vi "asap_rt_loop.vi"(4 "ASAP config":T1={"Calibration data"={"T1"=[], "K1"=[], "T2"=[], "K2"=[]}, "Block size"=0, "Tasks"={"Analog Input"="", "Counters"=[], "Digital out"=""}, "Light enables"=[], "Demodulator table"=[[[0.7378876894649258, 0.0906125472597644, -0.6039607285908369, -0.9832772754191942, -0.8493406206796001, -0.27206330946071283, 0.4472261971995385, 0.9330716049510009, 0.9318702757288254, 0.44424928196195224, -0.27526191405131173, -0.8510913000722428, -0.9826662061933111, -0.6013068779842613, 0.09392391656034481, 0.7401281017410278, 0.999998617584093], [0.9593453970107514, 0.1749709233028358, -0.8033628936873337, -0.8911502339509838, 0.008923213624955564, 0.8991050710898453, 0.7926080184909147, -0.19251348121496464, -0.9642293036540662, -0.6670744875896746, 0.36954793309667006, 0.9965178637479297, 0.5188245350812338, -0.5339978733406581, -0.9948712031832995, -0.3529066352920418, 0.6802631564678894]], [[0.6950304448649641, 0.029259796336992095, -0.6517839440467688, -0.9926080898406189, -0.8153085153483962, -0.21243243641618328, 0.5013295857114554, 0.9534065050307919, 0.907822232196422, 0.3883709446578477, -0.3338030496133024, -0.8817378051772073, -0.969421151739755, -0.5510839461787943, 0.15490925101319897, 0.7800425818962478, 0.9980075966531081], [0.9381204165433596, 0.10815294018097958, -0.8417045890860233, -0.8585129793585211, 0.07636026142185437, 0.9265863741042095, 0.749669912334455, -0.25827310590600655, -0.979914371470141, -0.615297735575794, 0.43139076953297817, 0.9998725601934042, 0.45997233240039587, -0.5898179378997009, -0.9857812880942376, -0.2889831231211053, 0.728159563799897]], [[-0.6523106754624476, 0.028565353817145308, 0.6945307778513148, 0.9979635224154992, 0.7804771064006715, 0.15559556021784737, -0.5505040934388046, -0.969250428253351, -0.8820653255595329, -0.33445785406592654, 0.38773065238112236, 0.9075306732447919, 0.953615867977217, 0.5019305868317728, -0.2117535089882616, -0.814906049621952, -0.9926921657471056], [-0.8972537749411549, -0.004712231334943897, 0.8930529304466017, 0.800848121012319, -0.17911548107307929, -0.9605254010675951, -0.6771705448338604, 0.3568436305984995, 0.9952883311784719, 0.5304327379276333, -0.5224198982706508, -0.9961579108878458, -0.3656316803152294, 0.6702057828807996, 0.9631045277016598, 0.18837947435655572, -0.7951686133781816]], [[-0.6100621017406637, 0.08296383725289572, 0.7326841328141306, 0.9999563780585607, 0.7452692276197674, 0.10156483182376178, -0.5951545948322141, -0.9812139372354715, -0.8550971038041967, -0.28263483236625087, 0.43735778093254624, 0.9290574326162326, 0.9358056736945096, 0.4540800426756246, -0.2646672723560626, -0.8452629914108203, -0.9846465037423504], [-0.8635658054477633, 0.06644929359614622, 0.9228038031878806, 0.756208806278458, -0.24866126331928293, -0.9778845315929664, -0.6231000231838354, 0.42240537195639455, 0.9996645751178765, 0.468772316125792, -0.5817649722709365, -0.9874022405026531, -0.2984811300725095, 0.7213132642049666, 0.9415151068455686, 0.1180255271232651, -0.8362980980464019]], [[0.5777399532793561, -0.12292948264806108, -0.7594319210118347, -0.9995244406514613, -0.717883028231008, -0.0615194781167083, 0.6269561424089901, 0.9881718380097269, 0.8335794576620439, 0.24387346683869626, -0.4731301243274189, -0.9431682286060581, -0.9208893384307617, -0.41792263714147493, 0.3031922273189156, 0.866046156382817, 0.9768394372642432], [0.817447755955057, -0.151248697507681, -0.9522824474358904, -0.6976889272021819, 0.3303090169266952, 0.992151723408322, 0.5541711388190733, -0.49812105893626973, -0.9982344623949164, -0.391781716958503, 0.6489701857141323, 0.9703235240149266, 0.21605063861728646, -0.777719411171446, -0.9093693817994032, -0.03296221490214164, 0.8799843348529361]], [[0.5316898836029471, -0.17765562828651216, -0.7942680705992896, -0.996286745386534, -0.6782615072995046, -0.006195858817183757, 0.6691039174680259, 0.9951433819294784, 0.8017357488499911, 0.18983635337997448, -0.5211542329290844, -0.9601116041437467, -0.8979078410494362, -0.36701219861201956, 0.3554572660433528, 0.8923843772058451, 0.9635027586436964], [0.7637113666149481, -0.2374642484157223, -0.9754052139040192, -0.632086784107158, 0.41191456619201, 0.9992990270168236, 0.4789372442711362, -0.5723376274536974, -0.9891629102916494, -0.3094780710033723, 0.7132704172557737, 0.9453420370266403, 0.12947999320562298, -0.8299136384717769, -0.8693286745034909, 0.05492737046661055, 0.9182951461013225]], [[-0.46766510452523, 0.24987476117295926, 0.8369844579156289, 0.9872031947765392, 0.6221194701815425, -0.06769952269503568, -0.7221805721079696, -0.9996962425675782, -0.7553883034308853, -0.11678114183164054, 0.5827836930773002, 0.9781458338214649, 0.862933293995299, 0.2972849646367805, -0.42354081435088226, -0.9232858418611823, -0.9410921262071124], [-0.6914685935131194, 0.33845772670298097, 0.9931957747140229, 0.5469531764674864, -0.5055997555832784, -0.9976835839369067, -0.38381192499528316, 0.6555241911872554, 0.9681964752983884, 0.20760041874903146, -0.7831255366749603, -0.9057385969172634, -0.024319329231539785, 0.8840584812667538, 0.8124368769318331, -0.15978992587511148, -0.9548858745902877]], [[-0.41626060082542315, 0.3049343375163701, 0.8669589900081666, 0.9764465114449328, 0.5762463682854527, -0.12474410208699359, -0.7606203759113978, -0.9994663787495118, -0.7166087568048619, -0.05969414412489584, 0.6283797471765561, 0.9884506172535718, 0.8325678935887533, 0.24209957785384775, -0.47474039981005334, -0.9437743555029069, -0.9201749293116044], [-0.631082800787636, 0.4130942080023554, 0.9993466668991985, 0.47780007230646987, -0.5733990296596044, -0.988971953675139, -0.3082464354209303, 0.71417743507813, 0.9449189867097926, 0.12819583587797975, -0.8306353845064933, -0.8686879369574549, 0.05622031910183376, 0.9188070421528223, 0.7628747613883726, -0.23872195854347844, -0.9756898279662225]]]}, 5 "error in":errorcluster, 6 "profile iterations":i32=10000, 7 "Stop after profile":bool, 8 "rt fifo":refnum<k33>) -> (0 "error out":errorcluster, 1 "total time histogram":T3(graph), 2 "mean time (uS)":dbl format="%.2f", 3 "cumulative times (uS)":dbl[][](graph))   [LabVIEW 2010]
uses:
  <vilib>/NI_Real-Time Target Support.lvlib
  <vilib>/Platform/TimedLoop/XDataNode/XDataNode.xnode
  <vilib>/Platform/TimedLoop/XDataNode/nitl_modes.ctl
  <vilib>/Platform/TimedLoop/XDataNode/XDNodeRunTimeDep.lvlib
  <vilib>/Platform/TimedLoop/XDataNode/wakeup.ctl
  <vilib>/Platform/TimedLoop/XDataNode/timing_clust.ctl
  <vilib>/Analysis/Matrix/Datatypes/RealMatrix.ctl
  <vilib>/Analysis/Matrix/NI_Matrix.lvlib
  initialization/configuration.ctl
panel:
  out "Num points":u64
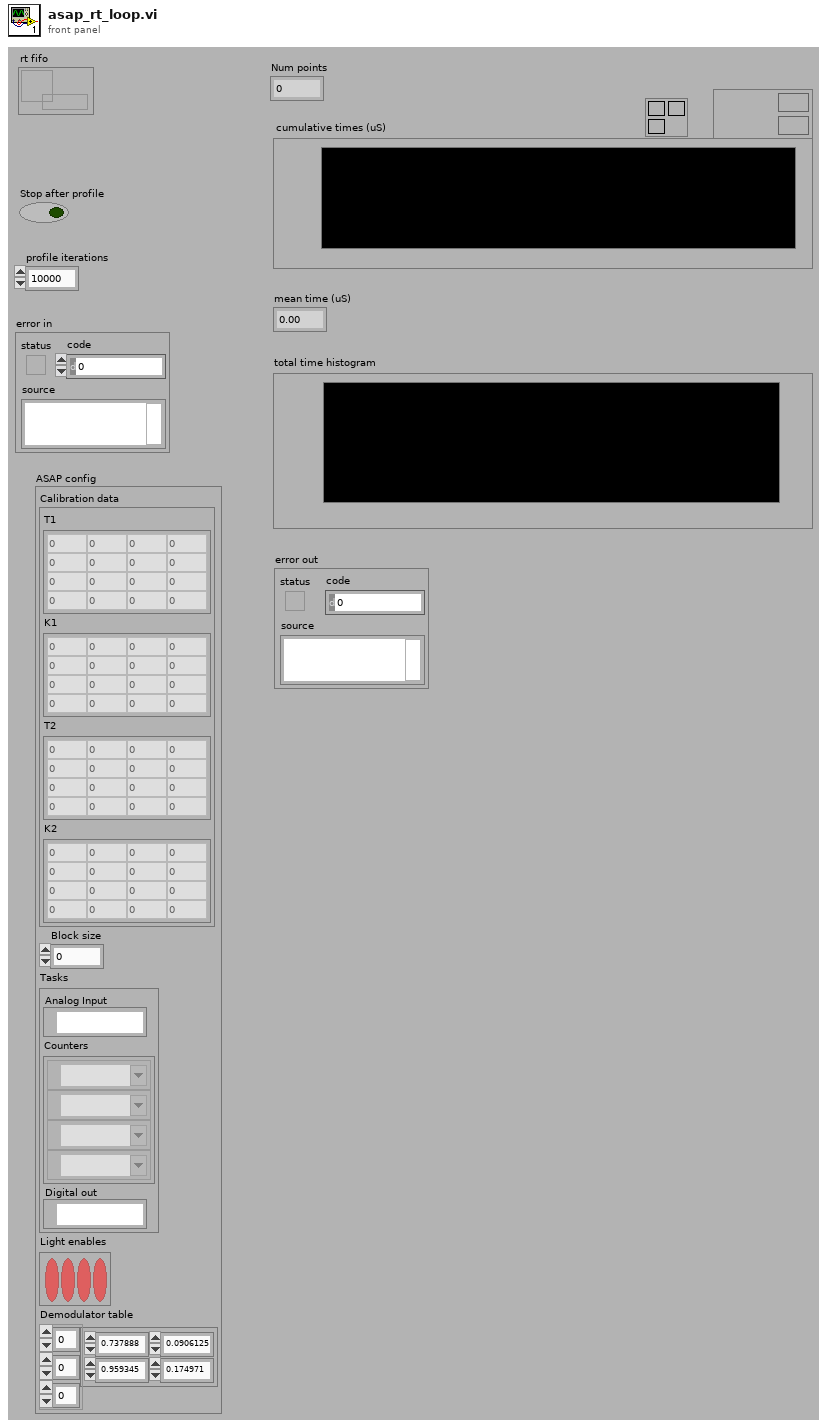
[diagram p1: front panel]
types:
  T1 = typedef "configuration.ctl" = cluster{"Calibration data":cluster{"T1":T2, "K1":T2, "T2":T2, "K2":T2}, "Block size":i32, "Tasks":cluster{"Analog Input":refnum<k21>, "Counters":refnum<k21>[], "Digital out":refnum<k21>}, "Light enables":bool[], "Demodulator table":dbl[][][]}
  T2 = typedef "NI_Matrix.lvlib/RealMatrix.ctl" = dbl[][]
  T3 = cluster{"X Values":dbl[], "Histogram: h(x)":i32[]}
  T4 = typedef "XDNodeRunTimeDep.lvlib/timing_clust.ctl" = cluster{"Expected End [f-1]":u64, "Actual End [f-1]":u64, "Finished Late? [f-1]":bool, "Expected End [i-1]":u64, "Actual End [i-1]":u64, "Finished Late? [i-1]":bool, "Expected Start [i]":u64, "Actual Start [i]":u64, "Expected Start [f]":u64, "Actual Start [f]":u64, "Source Name":string, "Structure Name":string, "Period":i64, "Deadline":i64, "Offset":i64, "Start":i64, "Priority":i32, "Timeout":i32, "Mode":T5, "Wakeup Reason":T6, "Error":errorcluster, "Source Type":string, "Secondary Source Type":string, "Global End Time":u64, "Global Start Time":u64, "Frame Duration":u64, "Iteration Duration":u64, "Assigned CPU":i32, "I/O Scan Engine Mode":u32}
  T5 = typedef "XDNodeRunTimeDep.lvlib/nitl_modes.ctl" = enum32{"No Change", "Process missed periods, maintain original phase", "Discard missed periods, maintain original phase", "Process missed periods, ignore original phase", "Discard missed periods, ignore original phase"}
  T6 = typedef "XDNodeRunTimeDep.lvlib/wakeup.ctl" = enum32{"Normal", "Aborted", "Asynchronous wakeup", "Timing source error", "Timed loop error", "Timeout"}
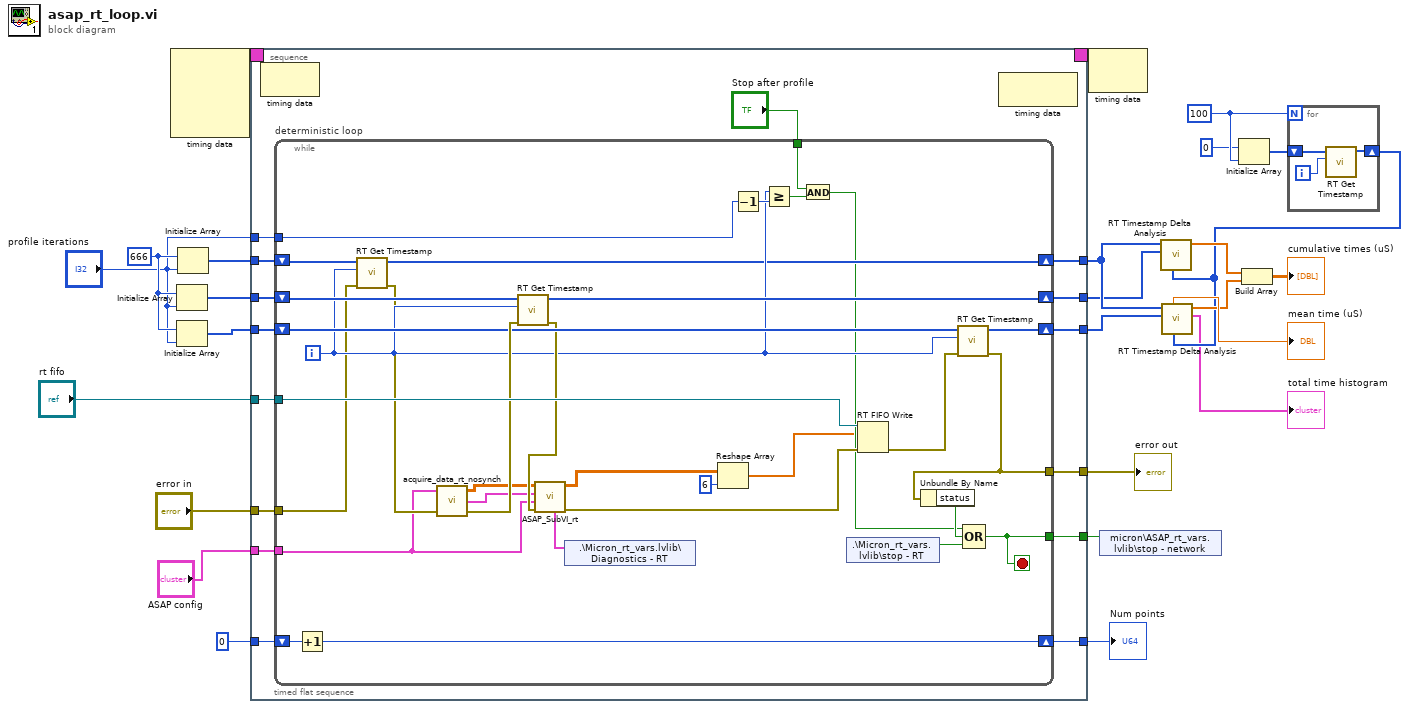
[diagram p0: block diagram]
diagram:
  w23 = u64 666 ("element")
  w11 = 100
  n1 = node-c288() -> (w4:T4)  [unwired: 4 in]
  n2 = Initialize Array(w23, "profile iterations") -> (w21:u64[])
  n3 = Initialize Array(w23, "profile iterations") -> (w22:u64[])
  n4 = Initialize Array(w23, "profile iterations") -> (w24:u64[])
  n5 = timed-sequence {
    timing: w4 -> [_]
    timing-out: [_] -> w3
    tunnel: "error in" -> [w40]
    tunnel: w24 -> [w39]
    tunnel: w22 -> [w38]
    tunnel: w21 -> [w37]
    tunnel: "profile iterations" -> [w36]
    tunnel: "ASAP config" -> [w35]
    tunnel: [w34] -> w18
    tunnel: [w33] -> w13
    tunnel: [w32] -> w12
    tunnel: [w31] -> w7
    tunnel: [w30] -> w6
    tunnel: "rt fifo" -> [w29]
    tunnel: u64 0 ("element") -> [w28]
    tunnel: [w27] -> w1
    n6 = timed-flat-sequence {
      tunnel: w40 -> [w55]
      tunnel: w39 -> [w54]
      tunnel: w38 -> [w53]
      tunnel: w37 -> [w52]
      tunnel: w36 -> [w51]
      tunnel: w35 -> [w50]
      tunnel: [w48] -> w34
      tunnel: [w47] -> w33
      tunnel: [w46] -> w32
      tunnel: [w45] -> w31
      tunnel: [w44] -> w30
      tunnel: w29 -> [w43]
      tunnel: w28 -> [w42]
      tunnel: [w41] -> w27
      n7 = node-c288() -> ()  [unwired: 1 in, 1 out]
      n8 = while "deterministic loop" {
        tunnel: w50 -> [w61]
        tunnel: [w69] -> w44
        tunnel: w55 -> [w74]
        tunnel: w43 -> [w87]
        tunnel: [w71] -> w45
        shift-right: [w83] -> w47
        shift-left: w52 -> [w84]
        shift-right: [w80] -> w46
        shift-left: w53 -> [w81]
        tunnel: w51 -> [w78]
        shift-right: [w72] -> w48
        shift-left: w54 -> [w76]
        tunnel: "Stop after profile" -> [w59]
        shift-right: [w56] -> w41
        shift-left: w42 -> [w57]
        i -> [w75]
        stop <- w71 stop-if-true
        n9 = Increment(x=w57) -> (x+1=w56:u64)
        n10 = call <vilib>:"RT Get Timestamp.vi"("error in (no error)"=w74, "iteration"=w75, "timestamp array in"=w76) -> ("error out"=w73:errorcluster, "timestamp array out"=w72:u64[])  [unwired: 7 in]
        n11 = call "acquire_data_rt_nosynch.vi"("error in"=w73, "Configuration"=w61) -> ("error out"=w82:errorcluster, "timestamp"=w66:cluster{"t0":timestamp, "dt":dbl}, "Data"=w65:sgl[][])  [unwired: 1 in]
        n12 = call <vilib>:"RT Get Timestamp.vi"("error in (no error)"=w82, "iteration"=w75, "timestamp array in"=w84) -> ("error out"=w77:errorcluster, "timestamp array out"=w83:u64[])  [unwired: 7 in]
        n13 = call "ASAP_SubVI_rt.vi"("error in"=w77, "Configuration"=w61, "Time in"=w66, "ADC data in"=w65) -> ("error out"=w68:errorcluster, "XYZ out"=w62:sgl[][], "Diagnostics"=w64:cluster{"Valid position":bool, "Message":string})  [unwired: 4 in, 1 out]
        n14 = shared-variable ".\\Micron_rt_vars.lvlib\\Diagnostics - RT"(w64) -> ()  [unwired: 1 in, 1 out]
        n15 = Reshape Array(w62, 6) -> (w58:sgl[])
        n16 = Decrement(x=w78) -> (x-1=w79:i32)
        n17 = Greater Or Equal?(x=w75, y=w79) -> (x >= y?=w60:bool)
        n18 = And(x=w59, y=w60) -> (x .and. y?=w67:bool)
        n19 = shared-variable ".\\Micron_rt_vars.lvlib\\stop - RT"() -> (w86:bool)  [unwired: 1 in, 1 out]
        n20 = RT FIFO Write(0:w87, 1:w58, 3:w68) -> (11:w70:errorcluster)  [unwired: 2 in, 3 out]
        n21 = call <vilib>:"RT Get Timestamp.vi"("error in (no error)"=w70, "iteration"=w75, "timestamp array in"=w81) -> ("error out"=w69:errorcluster, "timestamp array out"=w80:u64[])  [unwired: 7 in]
        n22 = Unbundle By Name(w69) -> ("status"=w85:bool)
        n23 = Compound Arithmetic op=OR(w67, w85, w86) -> (w71:bool)
      }
      n24 = node-c288() -> ()  [unwired: 1 in, 1 out]
    }
  }
  "error out" <- w6
  "Num points" <- w1
  n25 = node-c288(w3) -> ()  [unwired: 1 out]
  n26 = shared-variable "micron\\ASAP_rt_vars.lvlib\\stop - network"(w7) -> ()  [unwired: 1 in, 1 out]
  n27 = Initialize Array(u64 0 ("element"), w11) -> (w10:u64[])
  n28 = for {
    N: w11 -> [_]
    shift-right: [w90] -> w14
    shift-left: w10 -> [w92]
    i -> [w91]
    n29 = call <vilib>:"RT Get Timestamp.vi"("iteration"=w91, "timestamp array in"=w92) -> ("timestamp array out"=w90:u64[])  [unwired: 8 in, 1 out]
  }
  n30 = call "RT Timestamp Delta Analysis.vi"("calibration array"=w14, "timestamp array 2"=w13, "timestamp array 1"=w18) -> ("execution times (uS)"=w15:dbl[])  [unwired: 3 in, 5 out]
  n31 = call "RT Timestamp Delta Analysis.vi"("calibration array"=w14, "timestamp array 2"=w12, "timestamp array 1"=w18) -> ("execution histogram"=→"total time histogram":T3, "execution times (uS)"=w16:dbl[], "mean time (uS)"=→"mean time (uS)":dbl)  [unwired: 3 in, 3 out]
  n32 = Build Array(w15, w16) -> (→"cumulative times (uS)":dbl[][])
